vi "Addressing.vi"(8 "error in (no error)":errorcluster, 11 "Dali_usb_tridonics in":refnum<class "Dali_usb_tridonics.lvclass">) -> (0 "error out":errorcluster, 2 "Devices_Addresed":i32, 3 "Dali_usb_tridonics out":refnum<class "Dali_usb_tridonics.lvclass">)   [LabVIEW 2014, in "Driver_interaction.lvlib" / "Dali_usb_tridonics.lvclass"]
uses:
  Dali_usb_tridonics.lvclass
  _Driver_interaction/_Driver_interaction.lvclass
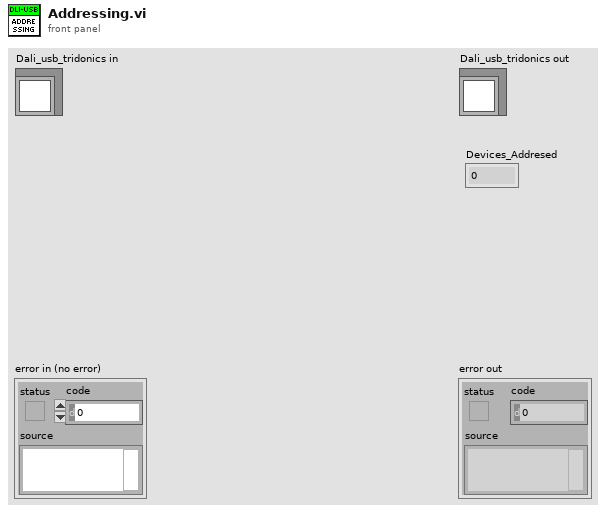
[diagram p1: front panel]
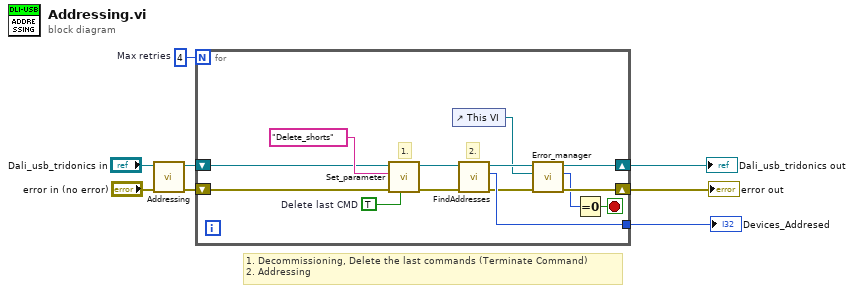
[diagram p0: block diagram]
diagram:
  w2 = 4  # Max retries
  # "1. Decommissioning, Delete the last commands (Terminate Command)\n2. Addressing"
  n1 = call-parent "Addressing.vi"("error in (no error)"="error in (no error)", "_Driver_interaction in"="Dali_usb_tridonics in") -> ("error out"=w5:errorcluster, "_Driver_interaction out"=w6:refnum<class "Dali_usb_tridonics.lvclass">)  [unwired: 7 in, 1 out]
  n2 = for {
    N: w2 -> [_]
    tunnel: [w13] -> w3
    shift-right: [w15] -> w4
    shift-left: w6 -> [w20]
    shift-right: [w14] -> w1
    shift-left: w5 -> [w19]
    stop <- w12 stop-if-true
    w21 = TRUE  # Delete last CMD
    # "2."
    # "1."
    n3 = call-dynamic "Set_parameter.vi"("Delete last CMD"=w21, "error in (no error)"=w19, "parameter"="Delete_shorts", "Dali_usb_tridonics in"=w20) -> ("error out"=w17:errorcluster, "Dali_usb_tridonics out"=w18:refnum<class "Dali_usb_tridonics.lvclass">)  [unwired: 6 in]
    n4 = control-ref of="This VI"() -> (w10:refnum<vi>)
    n5 = call-dynamic "FindAddresses.vi"("Dali_usb_tridonics in"=w18, "error in (no error)"=w17) -> ("Dali_usb_tridonics out"=w16:refnum<class "Dali_usb_tridonics.lvclass">, "Devices_Addressed"=w13:i32, "error out"=w9:errorcluster)  [unwired: 6 in]
    n6 = call-dynamic "Error_manager.vi"("error in (no error)"=w9, "Caller VI"=w10, "Dali_usb_tridonics in"=w16) -> ("error out"=w14:errorcluster, "code"=w11:i32, "Dali_usb_tridonics out"=w15:refnum<class "Dali_usb_tridonics.lvclass">)  [unwired: 4 in, 2 out]
    n7 = Equal To 0?(x=w11) -> (x = 0?=w12:bool)
  }
  "error out" <- w1
  "Dali_usb_tridonics out" <- w4
  "Devices_Addresed" <- w3
